vi "Untitled 1.vi"(8 "error in (no error)":errorcluster, 11 "WebSocket Service Actor in":refnum<class "WebSocket Service.lvclass">) -> (0 "error out":errorcluster, 3 "WebSocket Service Actor out":refnum<class "WebSocket Service.lvclass">)   [LabVIEW 2016, in "WebSocket Actors.lvlib" / "WebSocket Service.lvclass"]
uses:
  WebSocket Service.lvclass
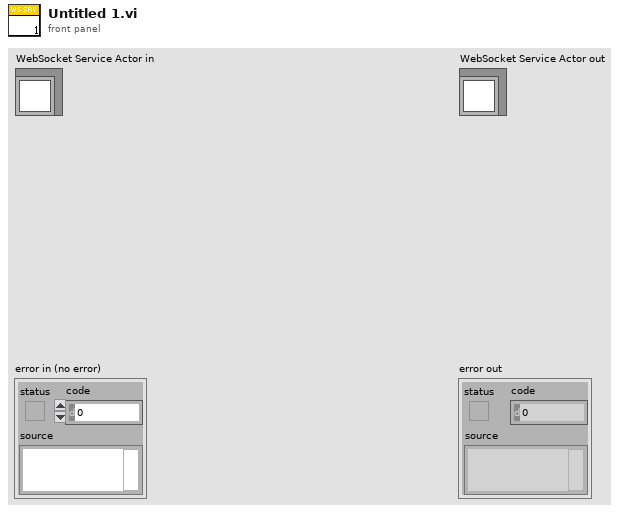
[diagram p1: front panel]
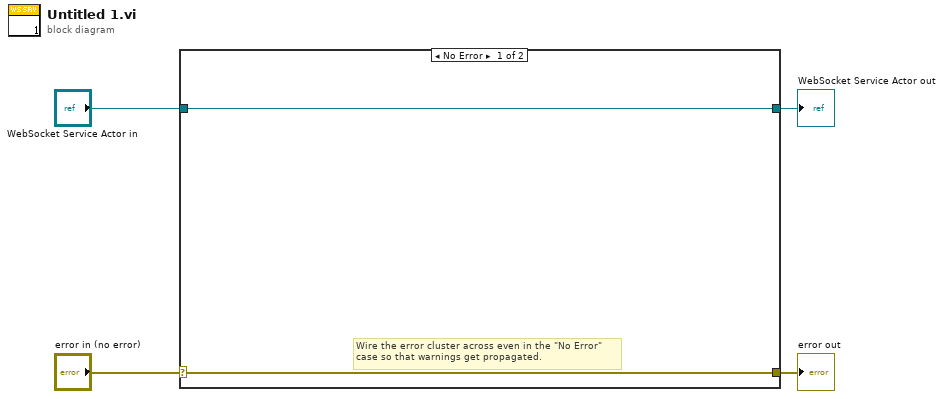
[diagram p0: block diagram]
diagram:
  n1 = case shown="No Error" "error in (no error)" {
    selector: "error in (no error)" -> [w5 w8]
    tunnel: [w5 w8] -> w3
    tunnel: [w6 w7] -> w1
    tunnel: "WebSocket Service Actor in" -> [w6 w7]
    frame No Error {
      # "Wire the error cluster across even in the \"No Error\"\ncase so that warnings get propagated."
    }
    frame Error {
    }
  }
  "error out" <- w3
  "WebSocket Service Actor out" <- w1
